vi "Compare Versions.vi"(7 "operator":T1, 8 "error in":errorcluster, 10 "version y":string, 11 "version x":string) -> (0 "error out":errorcluster, 3 "Satisfied?":bool)   [LabVIEW 2014, in "NIPM_API.lvlib"]
doc: "Executes a comparison operator on two version inputs"
uses:
  NIPM_API.lvlib
  _support/Version Comparison Operator.ctl
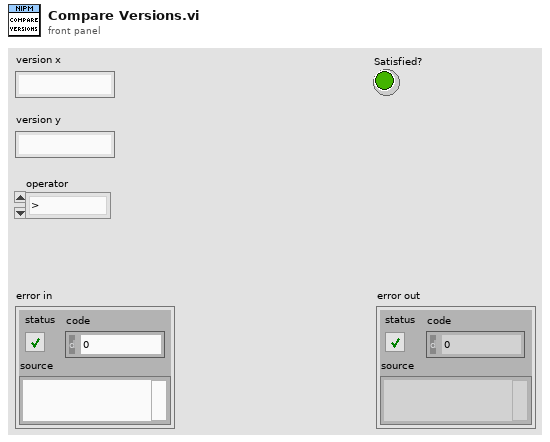
[diagram p1: front panel]
types:
  T1 = typedef "NIPM_API.lvlib/Version Comparison Operator.ctl" = enum16{">", ">=", "=", "!=", "<=", "<"}
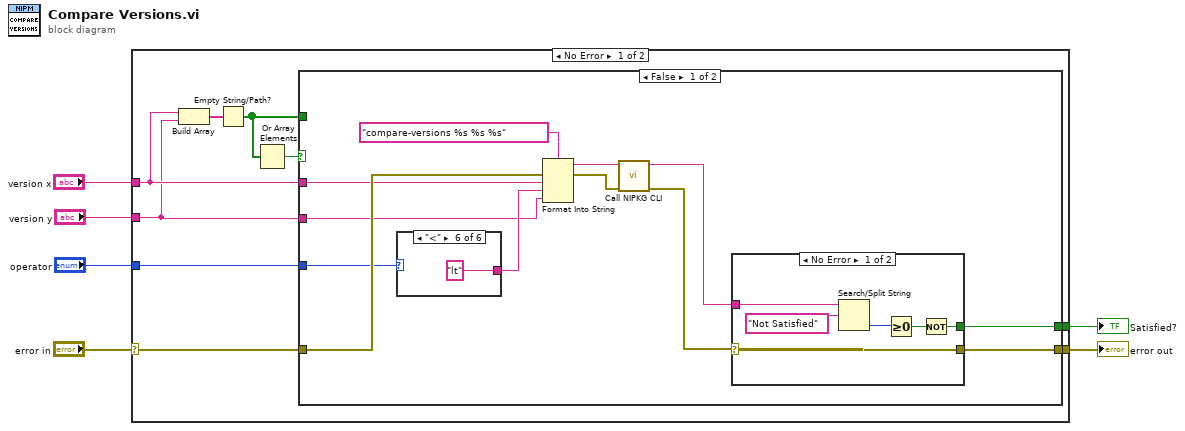
[diagram p0: block diagram]
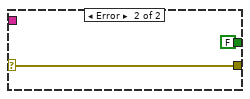
[diagram p2: hidden frame]
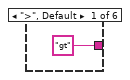
[diagram p3: hidden frame]
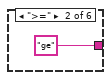
[diagram p4: hidden frame]
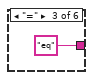
[diagram p5: hidden frame]
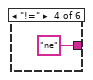
[diagram p6: hidden frame]
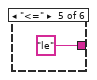
[diagram p7: hidden frame]
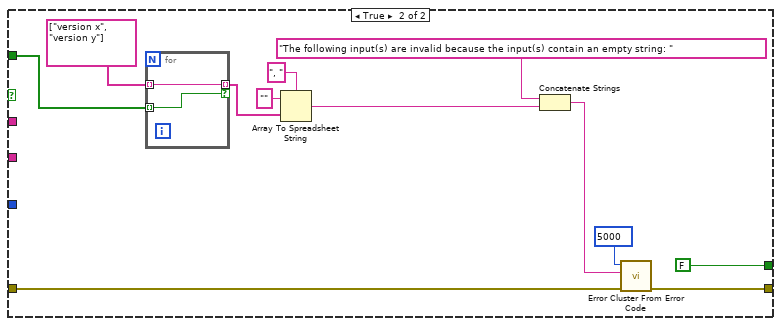
[diagram p8: hidden frame]
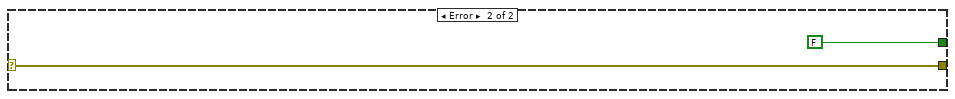
[diagram p9: hidden frame]
diagram:
  n1 = case shown="No Error" "error in" {
    selector: "error in" -> [w15 w57]
    tunnel: "operator" -> [w14 _]
    tunnel: "version x" -> [w11 _]
    tunnel: "version y" -> [w10 _]
    tunnel: [w13 w57] -> w2
    tunnel: [w12 FALSE] -> w1
    frame No Error {
      n2 = Build Array(w11, w10) -> (w9:string[])
      n3 = Empty String/Path?(string/path=w9) -> (empty?=w7:bool[])
      n4 = Or Array Elements(Boolean array=w7) -> (logical OR=w8:bool)
      n5 = case shown="False" w8 {
        tunnel: w15 -> [w26 w52]
        tunnel: w14 -> [w25 _]
        tunnel: [w23 w51] -> w13
        tunnel: [w22 FALSE] -> w12
        tunnel: w11 -> [w21 _]
        tunnel: w10 -> [w20 _]
        tunnel: w7 -> [_ w50]
        frame False {
          n6 = case shown="\"<\"" w25 {
            tunnel: ["gt" "ge" "eq" "ne" "le" "lt"] -> w24
            frame ">", Default {
            }
            frame ">=" {
            }
            frame "=" {
            }
            frame "!=" {
            }
            frame "<=" {
            }
            frame "<" {
            }
          }
          n7 = Format Into String(format string="compare-versions %s %s %s", error in=w26, w21, w24, w20) -> (resulting string=w18:string, error out=w17:errorcluster)  [unwired: 1 in]
          n8 = call "Call NIPKG CLI.vi"("error in (no error)"=w17, "command"=w18) -> ("error out"=w16:errorcluster, "command line standard output"=w19:string)  [unwired: 8 in]
          n9 = case shown="No Error" w16 {
            selector: w16 -> [w33 w35]
            tunnel: [w33 w35] -> w23
            tunnel: w19 -> [w31 _]
            tunnel: [w28 FALSE] -> w22
            frame No Error {
              n10 = Search/Split String(string=w31, search string/char (-)="Not Satisfied") -> (offset of match=w30:i32)  [unwired: 1 in, 2 out]
              n11 = Greater Or Equal To 0?(x=w30) -> (x >= 0?=w29:bool)
              n12 = Not(x=w29) -> (.not. x?=w28:bool)
            }
            frame Error {
            }
          }
        }
        frame True {
          n13 = for {
            tunnel: w50 -> [w54] mode=indexing
            tunnel: string[] ["version x", "version y"] -> [w55] mode=indexing
            tunnel: [w55] -> w48 mode=indexing if=w54
          }
          n14 = Array To Spreadsheet String(delimiter (Tab)=", ", array=w48, 3:"" ("format string")) -> (spreadsheet string=w44:string)
          n15 = Concatenate Strings("The following input(s) are invalid because the input(s) contain an empty string: ", w44) -> (w43:string)
          n16 = call <vilib>:"Error Cluster From Error Code.vi"("error in (no error)"=w52, "error message (\"\")"=w43, "error code (0)"=5000) -> ("error out"=w51:errorcluster)  [unwired: 6 in]
        }
      }
    }
    frame Error {
    }
  }
  "error out" <- w2
  "Satisfied?" <- w1
